vi "Configuration 1.2 JSON Flatten.vi"(8 "error in (no error)":errorcluster, 11 "configuration 1.2":T1={"plugins"=[{"name"="", "components"=[], "cycle timing"={"priority"=100, "decimation"=1, "offset"=0}, "threads"=[{"processor"=-2, "priority offset"=0, "settings"=[]}, {"processor"=-2, "priority offset"=0, "settings"=[]}, {"processor"=-2, "priority offset"=0, "settings"=[]}, {"processor"=-2, "priority offset"=0, "settings"=[]}], "transfer groups"=[{"name"="", "direction"=0, "cycle timing"={"priority"=100, "decimation"=1, "offset"=0}, "thread index"=0, "settings"=[], "transfers"=[{"name"="", "byte order"=0, "settings"=[], "channels"=[]}], "timeout behavior"=0}], "settings"=[]}]}) -> (0 "error out":errorcluster, 2 "file version":T2, 3 "configuration json":string)   [LabVIEW 2019, in "DSF Core.lvlib" / "Configuration Session.lvclass"]
uses:
  Configuration Session.lvclass
  Typedefs/DSF Version Info.ctl
  DSF Core.lvlib
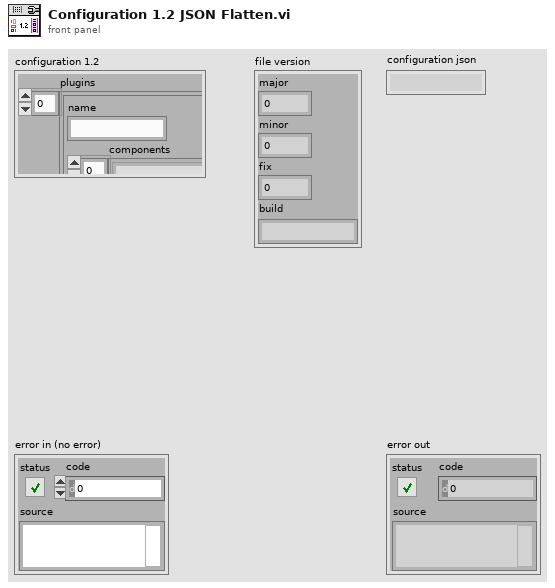
[diagram p1: front panel]
types:
  T1 = cluster{"plugins":cluster{"name":string, "components":string[], "cycle timing":cluster{"priority":u64, "decimation":u64, "offset":u64}, "threads":cluster{"processor":i32, "priority offset":i16, "settings":cluster{"component":string, "name":string, "values":cluster{"key":string, "value":string}[]}[]}[], "transfer groups":cluster{"name":string, "direction":u8, "cycle timing":cluster{"priority":u64, "decimation":u64, "offset":u64}, "thread index":i32, "settings":cluster{"component":string, "name":string, "values":cluster{"key":string, "value":string}[]}[], "transfers":cluster{"name":string, "byte order":u8, "settings":cluster{"component":string, "name":string, "values":cluster{"key":string, "value":string}[]}[], "channels":cluster{"string offset":u64, "name":string, "units":string, "engine data type":u8, "string data type":u8, "settings":cluster{"component":string, "name":string, "values":cluster{"key":string, "value":string}[]}[]}[]}[], "timeout behavior":u8}[], "settings":cluster{"component":string, "name":string, "values":cluster{"key":string, "value":string}[]}[]}[]}
  T2 = typedef "DSF Core.lvlib/DSF Version Info.ctl" = cluster{"major":u32, "minor":u32, "fix":u32, "build":string}
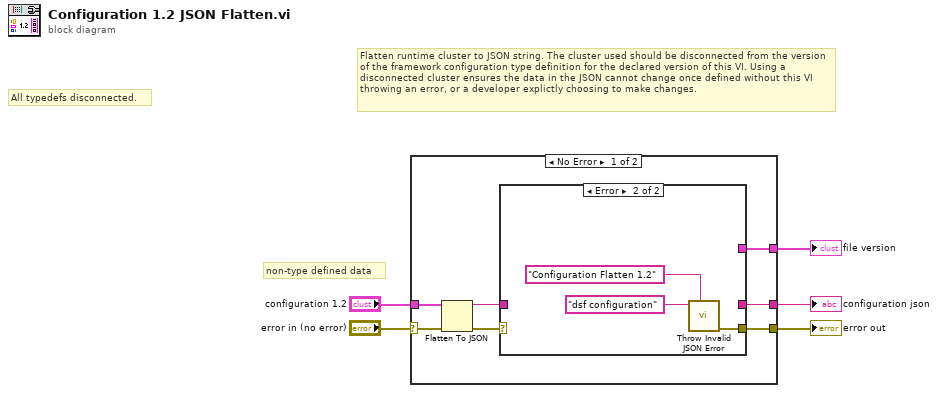
[diagram p0: block diagram]
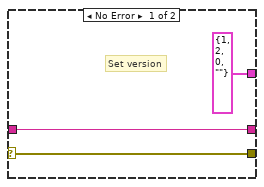
[diagram p2: hidden frame]
diagram:
  # "non-type defined data"
  # "All typedefs disconnected."
  # "Flatten runtime cluster to JSON string. The cluster used should be disconnected from the version of the framework configuration type definition for the declared version of this VI. Using a disconnected cluster ensures the data in the JSON cannot change once defined without this VI throwing an error, or a developer explictly choosing to make changes."
  n1 = case shown="No Error" "error in (no error)" {
    selector: "error in (no error)" -> [w9 w19]
    tunnel: [w11 w19] -> w5
    tunnel: "configuration 1.2" -> [w8 _]
    tunnel: [w7 _] -> w3
    tunnel: [w6 _] -> w2
    frame No Error {
      n2 = Flatten To JSON(anything=w8, error in (no error)=w9) -> (JSON string=w10:string, 11:w12:errorcluster)  [unwired: 1 in]
      n3 = case shown="Error" w12 {
        selector: w12 -> [w15 _]
        tunnel: [w15 w18] -> w11
        tunnel: w10 -> [w14 _]
        tunnel: [w14 _] -> w7
        tunnel: [T2 {"major"=1, "minor"=2, "fix"=0, "build"=""} ("json version") _] -> w6
        frame No Error {
          # "Set version"
        }
        frame Error {
          n4 = call "Throw Invalid JSON Error.vi"("error source vi name"="Configuration Flatten 1.2", "name"="dsf configuration") -> ("error out"=w18:errorcluster)  [unwired: 9 in]
        }
      }
    }
    frame Error {
    }
  }
  "configuration json" <- w3
  "error out" <- w5
  "file version" <- w2
